vi "Erase Selection.vi"(8 "error in (no error)":errorcluster, 9 "Shape in":refnum<data-value>[](array[refnum]), 10 "Selected in":i16[](array[numeric]), 11 "Image in":refnum<class "Image.lvclass">) -> (0 "error out":errorcluster, 1 "Shape out":refnum<data-value>[](array[refnum]), 2 "Selected out":i16[](array[numeric]), 3 "Image out":refnum<class "Image.lvclass">)   [LabVIEW 2015, in "LV Image Editor Framework.lvlib" / "Image Editor Handler.lvclass"]
uses:
  Image Editor Handler.lvclass
  Image/Image.lvclass
  Forms/Shape/Shape.lvclass
  Forms/Selection/Selection.lvclass
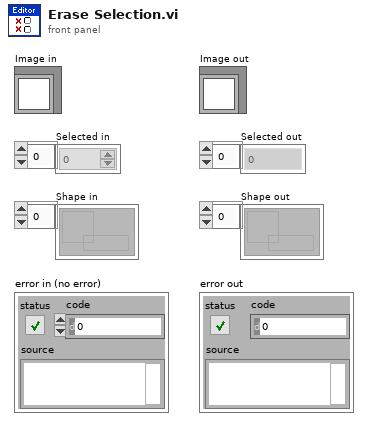
[diagram p1: front panel]
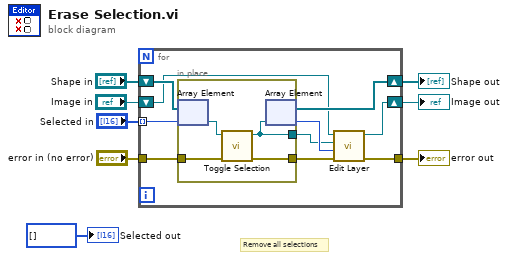
[diagram p0: block diagram]
diagram:
  # "Remove all selections"
  n1 = for {
    shift-right: [w12] -> w4
    shift-left: "Image in" -> [w13]
    tunnel: "Selected in" -> [w17] mode=indexing
    shift-right: [w14] -> w3
    shift-left: "Shape in" -> [w18]
    tunnel: "error in (no error)" -> [w11]
    tunnel: [w9] -> w8
    n2 = in-place {
      in-place-border: [w21] -> w15
      in-place-border: w11 -> [w20]
      in-place-border: [w19] -> w10
      n3 = in-place-array #1(w18, w17) -> (w22:refnum<data-value>)
      n4 = call "Toggle Selection.vi"("error in (no error)"=w20, "Shape"=w22) -> ("error out"=w19:errorcluster, "Shape"=w21:refnum<data-value>)  [unwired: 7 in, 1 out]
      n5 = in-place-array #1(w21) -> (w14:refnum<data-value>[], w16:i32)
    }
    n6 = call "Edit Layer.vi"("error in (no error)"=w10, "Layer Index"=w16, "ShapeRef"=w15, "Image in"=w13) -> ("error out"=w9:errorcluster, "Image out"=w12:refnum<class "Image.lvclass">)  [unwired: 6 in]
  }
  "error out" <- w8
  "Image out" <- w4
  "Shape out" <- w3
  "Selected out" <- i16[] [] ("Selected")
